vi "判断冲突.vi"(3 "OldVal":dbl, 4 "NewVal":dbl, 5 "Array":dbl[](array[numeric])) -> (2 "OutVal":dbl)   [LabVIEW 2013]
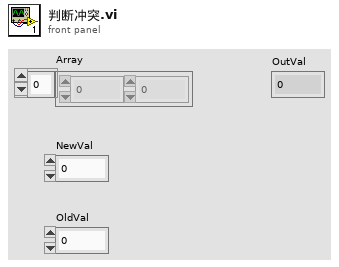
[diagram p1: front panel]
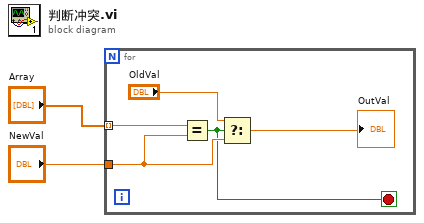
[diagram p0: block diagram]
diagram:
  n1 = for {
    tunnel: "Array" -> [w7] mode=indexing
    tunnel: "NewVal" -> [w4]
    stop <- w3 stop-if-true
    n2 = Equal?(x=w7, y=w4) -> (x = y?=w3:bool)
    n3 = Select(t="OldVal", s=w3, f=w4) -> (s? t:f=→"OutVal":dbl)
  }
